vi "Starting Positions.vi"(10 "Player Count":i32, 11 "Size":i32) -> (3 "Positions[]":cluster{i32, i32}[](array[cluster]))   [LabVIEW 2014, in "SquareBattle Arena.lvlib" / "SquareBattle Arena.lvclass"]
uses:
  SquareBattle Arena.lvclass
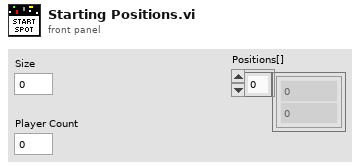
[diagram p1: front panel]
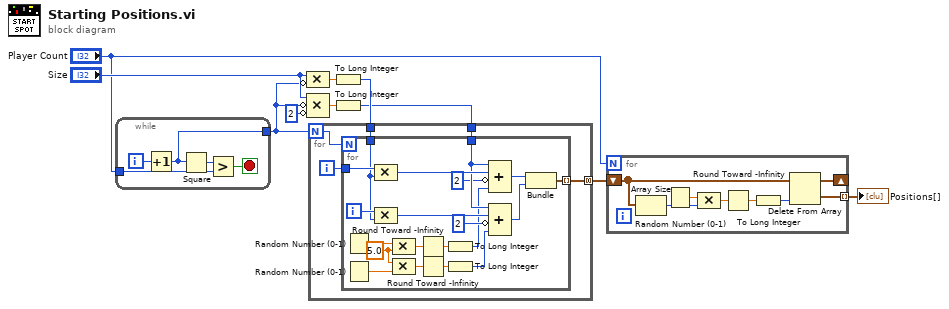
[diagram p0: block diagram]
diagram:
  n1 = while {
    tunnel: "Player Count" -> [w13]
    tunnel: [w12] -> w7
    i -> [w15]
    stop <- w14 stop-if-true
    n2 = Increment(x=w15) -> (x+1=w12:i32)
    n3 = Square(x=w12) -> (x^2=w11:i32)
    n4 = Greater?(x=w11, y=w13) -> (0:w14:bool)
  }
  n5 = Compound Arithmetic op=MULTIPLY("Size", invert w7) -> (w10:dbl)
  n6 = Compound Arithmetic op=MULTIPLY("Size", invert w7, invert 2 ("value")) -> (w9:dbl)
  n7 = To Long Integer(number=w10) -> (32bit integer=w5:i32)
  n8 = To Long Integer(number=w9) -> (32bit integer=w4:i32)
  n9 = for {
    N: w7 -> [w20]
    tunnel: w5 -> [w18]
    tunnel: w4 -> [w17]
    tunnel: [w16] -> w2 mode=concatenating
    i -> [w19]
    n10 = for {
      N: w20 -> [_]
      tunnel: w19 -> [w40]
      tunnel: w18 -> [w38]
      tunnel: w17 -> [w35]
      tunnel: [w32] -> w16 mode=indexing
      i -> [w39]
      w27 = 5.0 ("value")
      n11 = Random Number (0-1)() -> (number: 0 to 1=w29:dbl)
      n12 = Random Number (0-1)() -> (number: 0 to 1=w28:dbl)
      n13 = Compound Arithmetic op=MULTIPLY(w40, w38) -> (w37:i32)
      n14 = Compound Arithmetic op=MULTIPLY(w39, w38) -> (w36:i32)
      n15 = Compound Arithmetic op=MULTIPLY(w29, w27) -> (w26:dbl)
      n16 = Compound Arithmetic op=MULTIPLY(w27, w28) -> (w25:dbl)
      n17 = Round Toward -Infinity(1:w26) -> (0:w24:dbl)
      n18 = Round Toward -Infinity(1:w25) -> (0:w22:dbl)
      n19 = To Long Integer(number=w24) -> (32bit integer=w23:i32)
      n20 = To Long Integer(number=w22) -> (32bit integer=w21:i32)
      n21 = Compound Arithmetic op=ADD(w35, w37, invert 2 ("value"), w23) -> (w34:i32)
      n22 = Compound Arithmetic op=ADD(w35, w36, invert 2 ("value"), w21) -> (w33:i32)
      n23 = Bundle(w34, w33) -> (w32:cluster{i32, i32})  [unwired: 1 in]
    }
  }
  n24 = for {
    N: "Player Count" -> [_]
    shift-right: [w42] -> _
    shift-left: w2 -> [w44]
    tunnel: [w41] -> w1 mode=indexing
    n25 = Array Size(array=w44) -> (size(s)=w45:i32)
    n26 = Random Number (0-1)() -> (number: 0 to 1=w46:dbl)
    n27 = Compound Arithmetic op=MULTIPLY(w46, w45) -> (w47:dbl)
    n28 = Round Toward -Infinity(1:w47) -> (0:w48:dbl)
    n29 = To Long Integer(number=w48) -> (32bit integer=w43:i32)
    n30 = Delete From Array(array=w44, index=w43) -> (deleted portion=w41:cluster{i32, i32}, array with subset deleted=w42:cluster{i32, i32}[])  [unwired: 1 in]
  }
  "Positions[]" <- w1
